vi "GoBang_RemoveStones.vi"(1 "GameBoard in":u8[][](array[numeric])) -> (0 "GameBoard out":u8[][](array[numeric]))   [LabVIEW 2013, in "GoBang.lvlib"]
uses:
  GoBang.lvlib
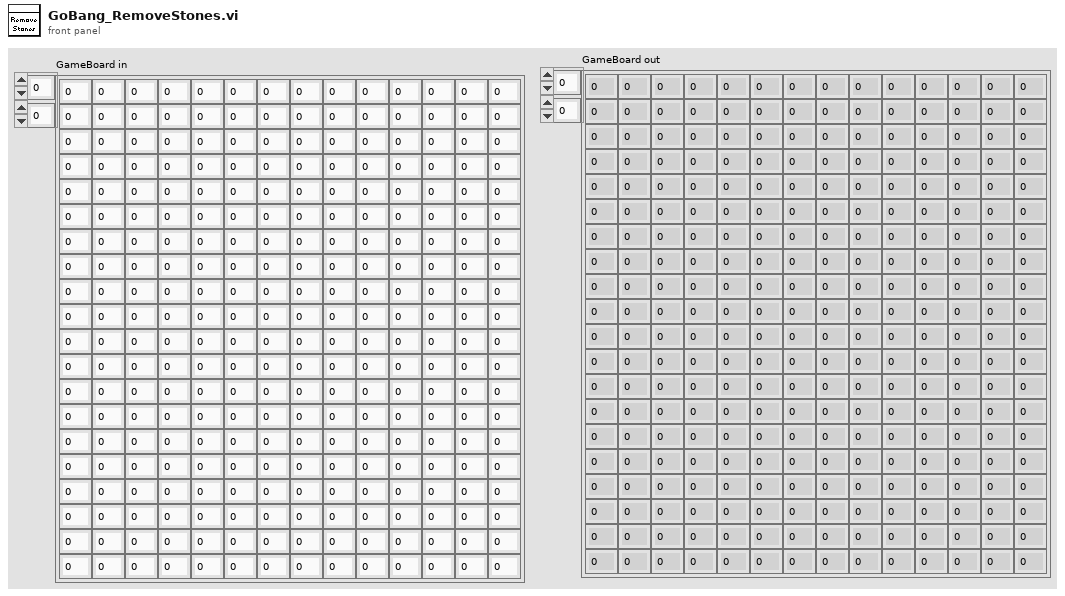
[diagram p1: front panel]
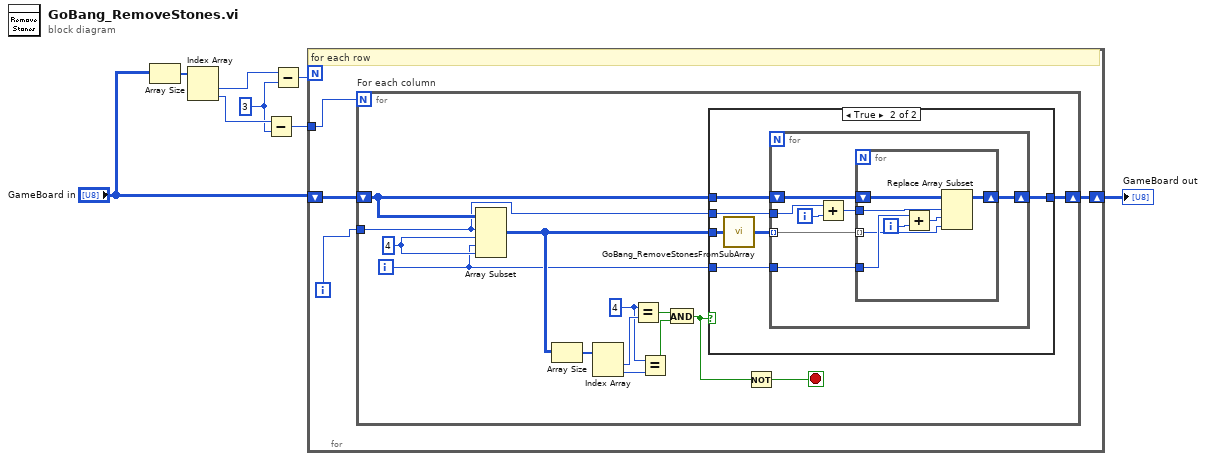
[diagram p0: block diagram]
diagram:
  w2 = 3 ("y")
  n1 = Array Size(array="GameBoard in") -> (size(s)=w7:i32[])
  n2 = Index Array(array=w7) -> (element #1=w6:i32, element #2=w4:i32)  [unwired: 2 in]
  n3 = Subtract(x=w4, y=w2) -> (x-y=w3:i32)
  n4 = Subtract(x=w6, y=w2) -> (x-y=w5:i32)
  n5 = for {
    N: w5 -> [_]
    tunnel: w3 -> [w10]
    shift-right: [w9] -> w1
    shift-left: "GameBoard in" -> [w12]
    i -> [w11]
    # "for each row"
    n6 = for "For each column" {
      N: w10 -> [_]
      tunnel: w11 -> [w15]
      shift-right: [w13] -> w9
      shift-left: w12 -> [w16]
      i -> [w14]
      stop <- w17 stop-if-true
      w21 = 4 ("x")
      w26 = 4 ("row N")
      n7 = Array Subset(array=w16, index (row)=w15, length (row)=w26, index (col)=w14, length (col)=w26) -> (w24:u8[][])
      n8 = Array Size(array=w24) -> (size(s)=w25:i32[])
      n9 = Index Array(array=w25) -> (element #1=w23:i32, element #2=w22:i32)  [unwired: 2 in]
      n10 = Equal?(x=w21, y=w23) -> (x = y?=w20:bool)
      n11 = Equal?(x=w21, y=w22) -> (x = y?=w19:bool)
      n12 = And(x=w20, y=w19) -> (x .and. y?=w18:bool)
      n13 = case shown="True" w18 {
        tunnel: w24 -> [_ w33]
        tunnel: w16 -> [w27 w31]
        tunnel: w15 -> [_ w30]
        tunnel: w14 -> [_ w29]
        tunnel: [w27 w28] -> w13
        frame False {
        }
        frame True {
          n14 = call "GoBang_RemoveStonesFromSubArray.vi"("4x4 array in"=w33) -> ("4x4 array out"=w32:u8[][])
          n15 = for {
            tunnel: w32 -> [w38] mode=indexing
            shift-right: [w39] -> w28
            shift-left: w31 -> [w40]
            tunnel: w30 -> [w37]
            tunnel: w29 -> [w34]
            i -> [w36]
            n16 = Add(x=w37, y=w36) -> (x+y=w35:i32)
            n17 = for {
              tunnel: w38 -> [w41] mode=indexing
              shift-right: [w46] -> w39
              shift-left: w40 -> [w47]
              tunnel: w35 -> [w43]
              tunnel: w34 -> [w42]
              i -> [w45]
              n18 = Add(x=w42, y=w45) -> (x+y=w44:i32)
              n19 = Replace Array Subset(array=w47, new element=w41, index (row)=w43, index (col)=w44) -> (w46:u8[][])
            }
          }
        }
      }
      n20 = Not(x=w18) -> (.not. x?=w17:bool)
    }
  }
  "GameBoard out" <- w1
